vi "DSF.Engine.Transceiver Thread.Transfer.Parse.vi"(8 "error in (no error)":errorcluster, 10 "Transfer":refnum<class "DSF.Engine.Transfer.lvclass">, 11 "Transceiver Thread in":refnum<class "DSF.Engine.Transceiver Thread.lvclass">) -> (0 "error out":errorcluster, 3 "Transceiver Thread out":refnum<class "DSF.Engine.Transceiver Thread.lvclass">)   [LabVIEW 2017, in "DSF.Engine.lvlib" / "DSF.Engine.Transceiver Thread.lvclass"]
uses:
  DSF.Engine.Transceiver Thread.lvclass
  Transfer/DSF.Engine.Transfer.lvclass
  DSF.Engine.Transceiver Thread.lvclass/DSF.Engine.Transceiver Thread.ctl
  Transfer/DSF.Engine.Transfer.lvclass/DSF.Engine.Transfer.ctl
  Buffer/DSF.Engine.Memory.Buffer.lvclass
  Pointer/DSF.Engine.Pointer.DBL.lvclass
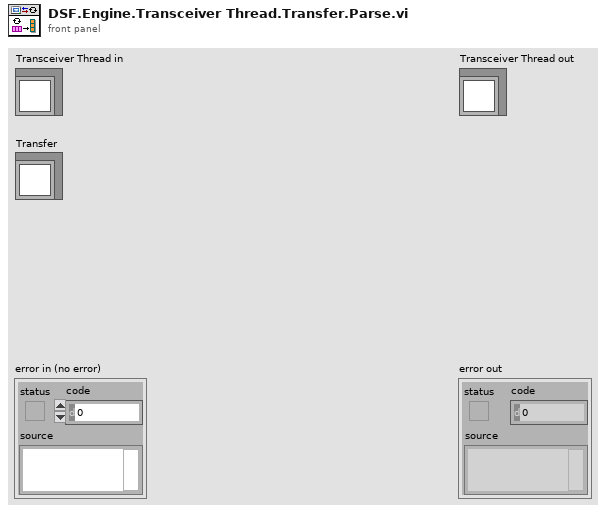
[diagram p1: front panel]
types:
  T1 = typedef "DSF.Engine.lvlib/DSF.Engine.Typedefs.Type Buffers.ctl" = cluster{"Bool":bool[], "SGL":sgl[], "DBL":dbl[], "I8":i8[], "I16":i16[], "I32":i32[], "I64":i64[], "U8":u8[], "U16":u16[], "U32":u32[], "U64":u64[]}
  T2 = typedef "DSF.Shared.lvlib/DSF.Shared.Typedefs.Configuration.Transfer.Channel Block Descriptor.ctl" = cluster{"First Channel Descriptor":T3, "count":u64, "vs channel index":u64}
  T3 = typedef "DSF.Shared.lvlib/DSF.Shared.Typedefs.Configuration.Transfer.Channel Descriptor.ctl" = cluster{"Channel Parameters":T4, "VS Channel Ref":T6}
  T4 = typedef "DSF.Shared.lvlib/DSF.Shared.Typedefs.Configuration.Transfer.Channel Parameters.ctl" = cluster{"offset":u64, "data type":T5}
  T5 = typedef "DSF.Shared.lvlib/DSF.Shared.Typedefs.Data Type.ctl" = enum8{"Bool", "SGL", "DBL", "I8", "I16", "I32", "I64", "U8", "U16", "U32", "U64"}
  T6 = typedef "Custom Device API.lvlib/Custom Device Item Ref.ctl" = u64
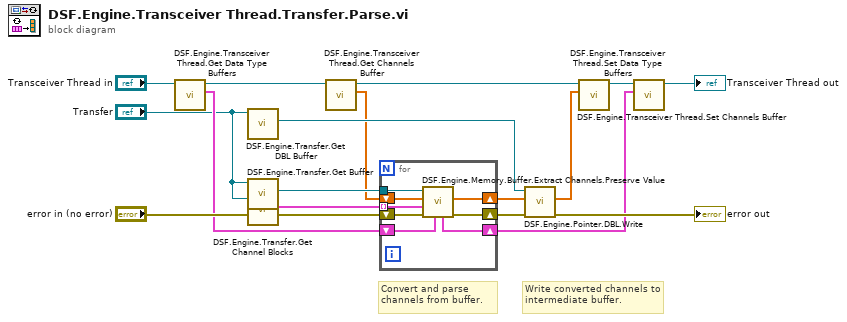
[diagram p0: block diagram]
diagram:
  # "Write converted channels to intermediate buffer."
  # "Convert and parse channels from buffer."
  n1 = call "DSF.Engine.Transceiver Thread.Get Data Type Buffers.vi"("Transceiver Thread in"="Transceiver Thread in") -> ("data type buffers"=w8:T1, "Transceiver Thread out"=w4:refnum<class "DSF.Engine.Transceiver Thread.lvclass">)  [unwired: 9 in]
  n2 = call "DSF.Engine.Transfer.Get DBL Buffer.vi"("Transfer in"="Transfer") -> ("DBL Buffer"=w13:refnum<class "DSF.Engine.Pointer.DBL.lvclass">)  [unwired: 9 in, 1 out]
  n3 = call "DSF.Engine.Transfer.Get Buffer.vi"("Transfer in"="Transfer") -> ("Buffer"=w16:refnum<class "DSF.Engine.Memory.Buffer.lvclass">)  [unwired: 9 in, 1 out]
  n4 = call "DSF.Engine.Transfer.Get Channel Blocks.vi"("Transfer in"="Transfer") -> ("Channel Blocks"=w1:T2[])  [unwired: 9 in, 1 out]
  n5 = call "DSF.Engine.Transceiver Thread.Get Channels Buffer.vi"("Transceiver Thread in"=w4) -> ("channels buffer"=w11:dbl[], "Transceiver Thread out"=w9:refnum<class "DSF.Engine.Transceiver Thread.lvclass">)  [unwired: 9 in]
  n6 = for {
    shift-right: [w24] -> w14
    shift-left: w11 -> [w21]
    shift-right: [w25] -> w15
    shift-left: "error in (no error)" -> [w23]
    tunnel: w16 -> [w20]
    tunnel: w1 -> [w22] mode=indexing
    shift-right: [w19] -> w7
    shift-left: w8 -> [w18]
    n7 = call "DSF.Engine.Memory.Buffer.Extract Channels.Preserve Value.vi"("Data Type Buffers in"=w18, "error in (no error)"=w23, "Channel Block"=w22, "VS Channels Array in"=w21, "Buffer in"=w20) -> ("error out"=w25:errorcluster, "VS Channels Array out"=w24:dbl[], "Data Type Buffers out"=w19:T1)  [unwired: 3 in, 1 out]
  }
  n8 = call "DSF.Engine.Pointer.DBL.Write.vi"("error in (no error)"=w15, "buffer in"=w14, "DBL Pointer in"=w13) -> ("error out"=→"error out":errorcluster, "buffer out"=w10:dbl[])  [unwired: 6 in, 1 out]
  n9 = call "DSF.Engine.Transceiver Thread.Set Channels Buffer.vi"("channels buffer"=w10, "Transceiver Thread in"=w9) -> ("Transceiver Thread out"=w3:refnum<class "DSF.Engine.Transceiver Thread.lvclass">)  [unwired: 9 in]
  n10 = call "DSF.Engine.Transceiver Thread.Set Data Type Buffers.vi"("data type buffers"=w7, "Transceiver Thread in"=w3) -> ("Transceiver Thread out"=→"Transceiver Thread out":refnum<class "DSF.Engine.Transceiver Thread.lvclass">)  [unwired: 9 in]
